vi "PH_PPPA_PowerUnit.src Switch GD Channel on.vi"(0 "i ref in":refnum<vi>, 5 "error in (no error)":errorcluster) -> (14 "i ref out":refnum<vi>, 19 "error out":errorcluster)   [LabVIEW 2014, in "PH_PPPA_PowerUnit.lvlib"]
doc: "This is the action VI of the _StateTrigger event case. If \n\n2 (triggered): if SM state = \"Switch GD Channel on\", a state change request is send to SM to get \"Close Ross Relais\"."
uses:
  PH_PPPA_PowerUnit.lvlib
  PH_Basics/PH_PowerUnit_BaseClass/PH_PowerUnit_BaseClass.SM States.ctl
  PH_Basics/PH_PowerUnit_BaseClass/PH_PowerUnit_BaseClass.lvlib
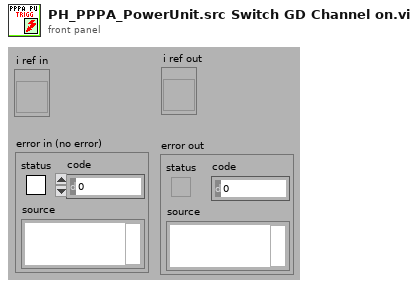
[diagram p1: front panel]
types:
  T1 = typedef "PH_PPPA_PowerUnit.lvlib/PH_PPPA_PowerUnit.i attribute.ctl" = cluster{"GUI Refs":cluster{"Ignitron":refnum<vi>, "Rossrelais":refnum<vi>, "Set Voltage":refnum<vi>, "PSU":refnum<vi>, "EOC":refnum<vi>, "Trigger":refnum<vi>}, "Ignitron":T2, "PSU":T4, "Dump Ross Relais":T5, "Trigger":cluster{"State Device":T3, "linked?":bool}, "Timing Settings":cluster{"Prdc Fast?":bool, "Default Value Periodic Interval":i32, "Mercury on since":dbl, "Warm up Time Mercury [s]":dbl}, "Set Voltage [V]":dbl, "19er Ignitionbox":string}
  T2 = typedef "PH_PP_Common.lvlib/PH_PP_Common.Ignitron Attributes.ctl" = cluster{"State Device":T3, "linked?":bool}
  T3 = typedef "PH_StatusHandler.lvlib/PH_StatusHandler.Status.ctl" = i16
  T4 = typedef "PH_PP_Common.lvlib/PH_PP_Common.PSU Attributes.ctl" = cluster{"lower limit [V]":dbl, "upper limit [V]":dbl, "Voltage set":bool, "State Device":T3, "linked?":bool}
  T5 = typedef "PH_PP_Common.lvlib/PH_PP_Common.Ross Relais Attributes.ctl" = cluster{"State Device":T3, "linked?":bool}
  T6 = typedef "PH_PowerUnit_BaseClass.lvlib/PH_PowerUnit_BaseClass.SM States.ctl" = enum16{".", "Stand by", "Switch PU on", "Configure", "Set Default Voltage", "Set STANDBY", "Set READY", "Wait for Shot Cmd", "Open Dump Rods", "Open Ross Relais", "Close Ross Relais", "Switch PSU on", "Switch PSU off", "Charge", "Switch GD Channel on", "Close Dump Rods", "Rods-TO", "RR-TO", "PSU-TO", "Trigger-TO"}
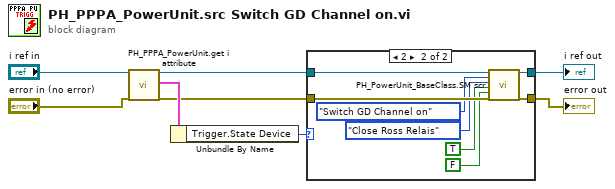
[diagram p0: block diagram]
diagram:
  n1 = call "PH_PPPA_PowerUnit.get i attribute.vi"("i ref in"="i ref in", "error in (no error)"="error in (no error)") -> ("i ref out"=w5:refnum<vi>, "i attribute"=w8:T1, "error out"=w4:errorcluster)  [unwired: 15 in]
  n2 = Unbundle By Name(w8) -> ("Trigger.State Device"=w3:T3)
  n3 = case shown="2" w3 {
    tunnel: w5 -> [w10 w17]
    tunnel: w4 -> [w9 w18]
    tunnel: [w9 w13] -> w1
    tunnel: [w10 w14] -> w2
    frame Default {
    }
    frame 2 {
      n4 = call "PH_PowerUnit_BaseClass.SM scr.vi"("VI in"=w17, "Current SM State (condition)"=PH_PowerUnit_BaseClass.SM_States."Switch GD Channel on", "Wanted SM State"=PH_PowerUnit_BaseClass.SM_States."Close Ross Relais", "Further change condition"=TRUE, "PU in use is condition? (true)"=FALSE, "error in (no error)"=w18) -> ("VI out"=w14:refnum<vi>, "error out"=w13:errorcluster)  [unwired: 12 in]
    }
  }
  "error out" <- w1
  "i ref out" <- w2
